vi "setValueDH.vi"(7 "TableName":string, 8 "error in (no error)":errorcluster, 9 "Value":string, 10 "ItemName":string, 11 "DataHandler in":refnum<class "DataHandler.lvclass">) -> (0 "error out":errorcluster, 3 "DataHandler out":refnum<class "DataHandler.lvclass">)   [LabVIEW 2017, in "DataHandler.lvclass"]
uses:
  DataHandler.lvclass
  DataHandler.lvclass/DataHandler.ctl
  <vilib>/drjdpowell/SQLite Library/SQL Connection/Execute SQL (No results).vi
  <vilib>/drjdpowell/SQLite Library/Transaction Helpers/Transaction.lvlib
  <vilib>/drjdpowell/SQLite Library/SQLite.lvlib
  <vilib>/drjdpowell/SQLite Library/SQL Connection/Connection.lvclass
panel:
  out "concatenated string":string
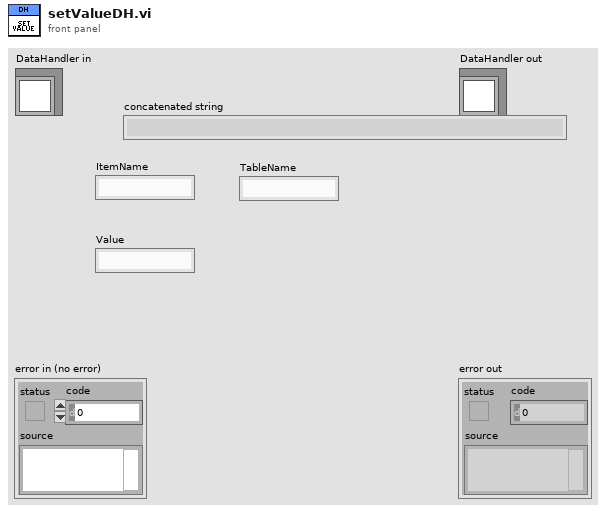
[diagram p1: front panel]
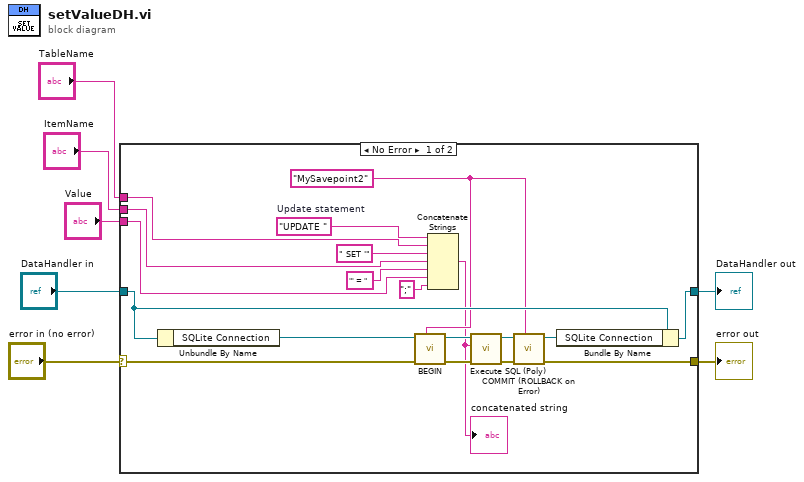
[diagram p0: block diagram]
diagram:
  n1 = case shown="No Error" "error in (no error)" {
    selector: "error in (no error)" -> [w21 w28]
    tunnel: [w20 w28] -> w6
    tunnel: [w25 w27] -> w4
    tunnel: "DataHandler in" -> [w26 w27]
    tunnel: "Value" -> [w9 _]
    tunnel: "ItemName" -> [w16 _]
    tunnel: "TableName" -> [w17 _]
    frame No Error {
      w14 = "MySavepoint2" ("Savepoint name")
      w19 = "UPDATE "  # Update statement
      n2 = Unbundle By Name(w26) -> ("SQLite Connection"=w24:refnum<class "Connection.lvclass">)
      n3 = call <vilib>:"BEGIN.vi"("Savepoint name"=w14, "error in (no error)"=w21, "Connection in"=w24) -> ("error out"=w11:errorcluster, "Connection out"=w15:refnum<class "Connection.lvclass">)  [unwired: 7 in]
      n4 = Concatenate Strings(w19, w17, " SET '" ("string"), w16, "' = " ("string"), w9, ";" ("string")) -> (w10:string)
      "concatenated string" <- w10
      n5 = call-poly <vilib>:"Execute SQL (Poly).vi"("error in (no error)"=w11, "SQL"=w10, "SQLite Connection in"=w15) -> ("error out"=w12:errorcluster, "SQLite Connection out"=w13:refnum<class "Connection.lvclass">)  [unwired: 7 in]
      n6 = call <vilib>:"COMMIT (ROLLBACK on Error).vi"("Savepoint name"=w14, "error in (no error)"=w12, "Connection in"=w13) -> ("error out"=w20:errorcluster, "Connection out"=w23:refnum<class "Connection.lvclass">)  [unwired: 7 in]
      n7 = Bundle By Name(cluster=w26, "SQLite Connection"=w23) -> (w25:refnum<class "DataHandler.lvclass">)
    }
    frame Error {
    }
  }
  "error out" <- w6
  "DataHandler out" <- w4
